vi "Execute.vi"(8 "error in (no error)":errorcluster, 11 "CIFTemplatePlugin in":refnum<class "TemplatePlugin.lvclass">) -> (0 "error out":errorcluster, 3 "CIFTemplatePlugin out":refnum<class "TemplatePlugin.lvclass">)   [LabVIEW 2021, in "TemplatePlugin.lvclass"]
uses:
  TemplatePlugin.lvclass
  D:/dev/CIF-LVCore/src/CIFCore/Class/CIFCorePlugin.lvclass
  CIF-LVCore/src/CIFCore/Class/Typedef/Energized States.ctl
  CIF-LVCore/src/CIFCore/Class/CIFCorePlugin.lvclass/CIFCorePlugin.ctl
  TemplatePlugin.lvclass/TemplatePlugin.ctl
  CIF-LVCore/src/CIFCore/Class/Channel RW/Read U64.vi
  CIF-LVCore/src/CIFCore/Class/Channel RW/Write U64.vi
  CIF-LVCore/src/CIFCore/Class/Channel RW/Write Double.vi
  CIF-LVCore/src/CIFCore/Class/Channel RW/Read Double.vi
  CIF-LVCore/src/CIFCore/Class/Accessors/Monitor/Write Double 1.vi
  CIF-LVCore/src/CIFCore/Class/Accessors/Monitor/Write U64 1.vi
  CIF-LVCore/src/CIFCore/Class/Accessors/Monitor/Write U64 2.vi
  CIF-LVCore/src/CIFCore/Class/Accessors/Monitor/Write I64 1.vi
  CIF-LVCore/src/CIFCore/Class/Accessors/Monitor/Write I64 2.vi
  CIF-LVCore/src/CIFCore/Class/Accessors/Timestamps/Write Execute TS.vi
  CIF-LVCore/src/CIFCore/Class/Accessors/Timestamps/Write Sleep TS.vi
  <vilib>/Utility/error.llb/Clear Errors.vi
  <vilib>/CIF Foundation/CIF Utilities/Time/System Time/Sleep Until Future Time.vi
  CIF-LVCore/src/CIFCore/Class/Accessors/Read Sleep Limits (ns).vi
  CIF-LVCore/src/CIFCore/Class/Accessors/Timestamps/Write Target Wake TS.vi
  CIF-LVCore/src/CIFCore/Class/SubVIs/Start Running.vi
  CIF-LVCore/src/CIFCore/Class/Accessors/Read Plugin Name.vi
  <vilib>/CIF Foundation/CIF Utilities/Time/System Time/Get System Time.vi
  CIF-LVCore/src/CIFCore/Common/Utilities/Add Error.vi
  CIF-LVCore/src/CIFCore/Class/Accessors/Timestamps/Read Running TS.vi
  CIF-LVCore/src/CIFCore/Class/Benchmarking/Reset Delay.vi
  CIF-LVCore/src/CIFCore/Class/Accessors/Read Running Internal Data.vi
  CIF-LVCore/src/CIFCore/Class/Accessors/Read Timing Override.vi
  CIF-LVCore/src/CIFCore/Class/Accessors/Read Common Config.vi
  <vilib>/CIF Foundation/CIF Utilities/Time/SubVIs/Add Error.vi
  <vilib>/CIF Foundation/CIF Utilities/Time/System Time/LabVIEW Time to TAI Time.vi
  <vilib>/CIF Foundation/CIF Utilities/Errors/Append Error Location.vi
  <vilib>/CIF Foundation/CIF Channels Core/CIFChannels/CIFChannels.lvclass
  CIF-LVCore/src/CIFCore/Class/CIFCorePlugin.lvclass
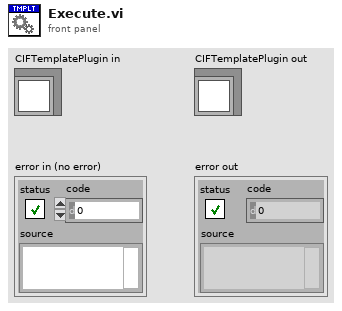
[diagram p1: front panel]
types:
  T1 = typedef "CIFCorePlugin.lvclass/Energized States.ctl" = enum16{"Listen", "Prepare", "Execute", "Housekeep", "Cleanup", "Destroy"}
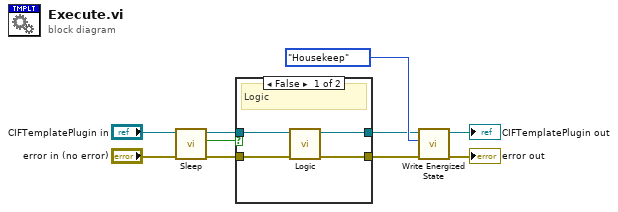
[diagram p0: block diagram]
diagram:
  n1 = call "Sleep.vi"("error in (no error)"="error in (no error)", "CIFCorePlugin in"="CIFTemplatePlugin in") -> ("error out"=w7:errorcluster, "Housekeep only"=w8:bool, "CIFCorePlugin out"=w6:refnum<class "TemplatePlugin.lvclass">)  [unwired: 7 in]
  n2 = case shown="False" w8 {
    tunnel: [w12 w15] -> w1
    tunnel: [w13 w16] -> w9
    tunnel: w6 -> [w14 w16]
    tunnel: w7 -> [w11 w15]
    frame False {
      # "Logic"
      n3 = call "Logic.vi"("error in (no error)"=w11, "CIFTemplatePlugin in"=w14) -> ("error out"=w12:errorcluster, "CIFTemplatePlugin out"=w13:refnum<class "TemplatePlugin.lvclass">)  [unwired: 8 in]
    }
    frame True {
      # "Housekeep only"
    }
  }
  n4 = call "Write Energized State.vi"("error in (no error)"=w1, "Energized State"=Energized_States."Housekeep", "CIFCorePlugin in"=w9) -> ("error out"=→"error out":errorcluster, "CIFCorePlugin out"=→"CIFTemplatePlugin out":refnum<class "TemplatePlugin.lvclass">)  [unwired: 7 in]
